vi "pupilometria_IR.vi"() -> ()   [LabVIEW 2024]
uses:
  <vilib>/vision/NI_Vision_Development_Module.lvlib
panel:
  out "Gray Image":T1(plugin-control)
  out "ROI manual":T1(plugin-control)
  out "error out":errorcluster
  in  "stop":bool
  out "Image Out":T1(plugin-control)
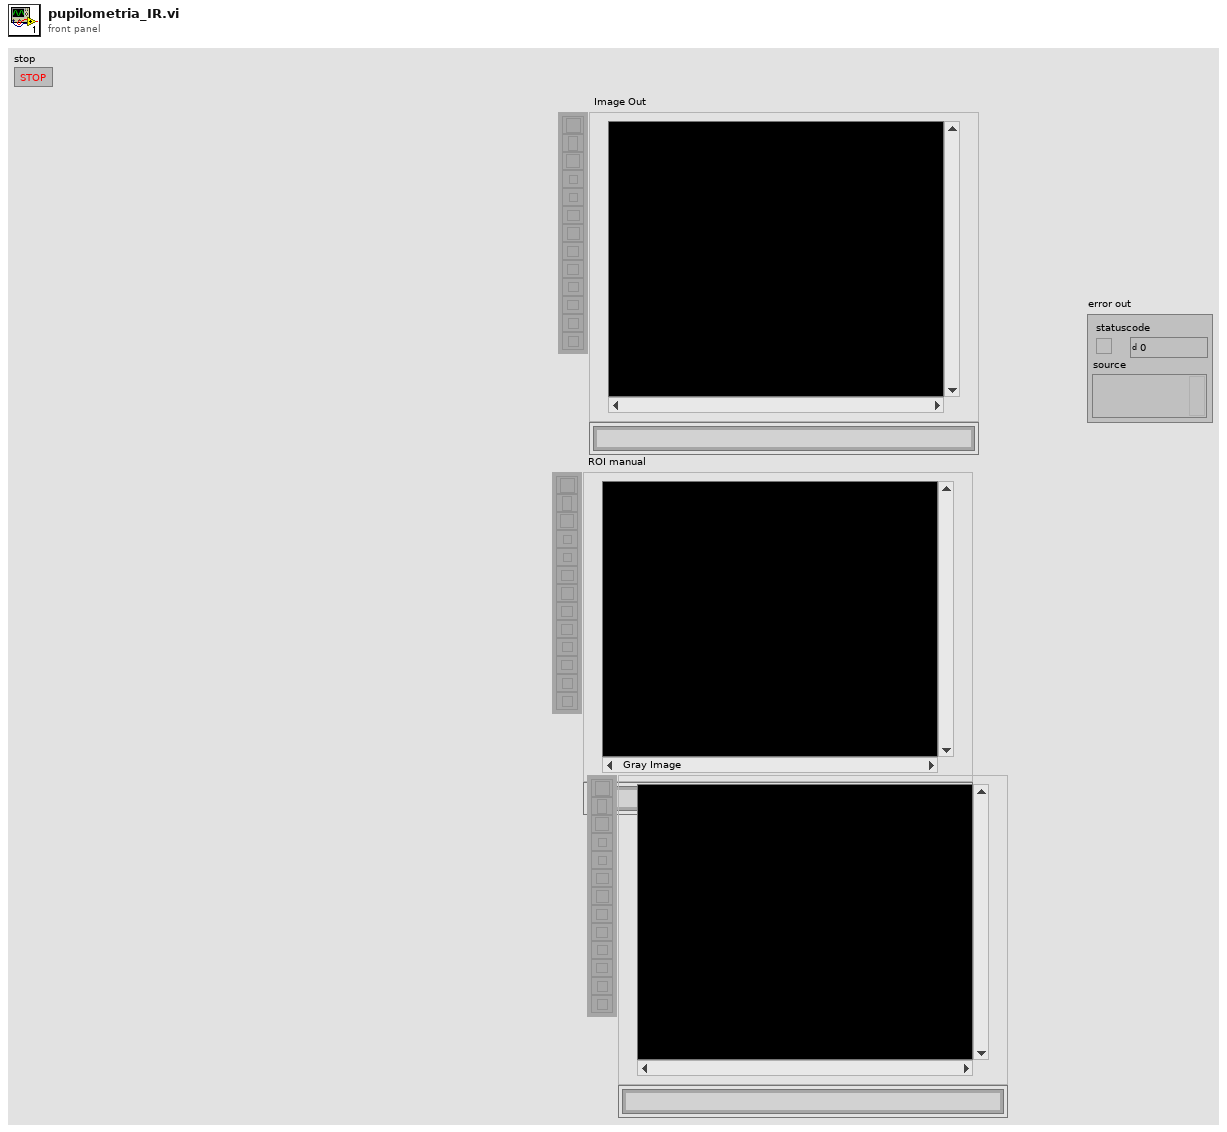
[diagram p1: front panel]
types:
  T1 = typedef "IMAQ Image.ctl" = refnum<image>
  T2 = typedef "Image Type" = u32
  T3 = cluster{"Global Rectangle":i32[], "Contours":cluster{"Contour Type":u32, "ROI Type":u32, "Points":i32[]}[]}
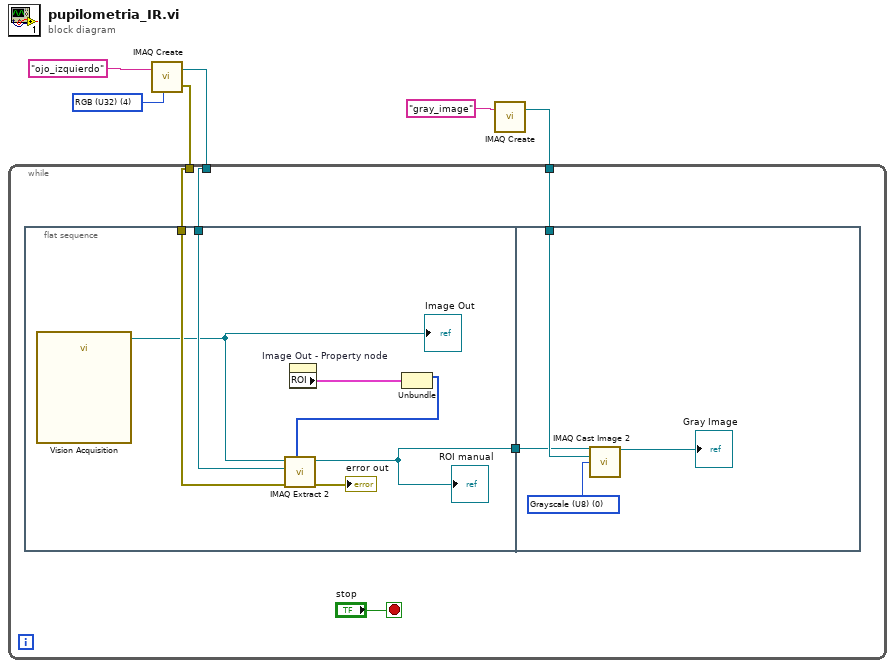
[diagram p0: block diagram]
diagram:
  w5 = T2 4 items=["Grayscale (U8)", "Grayscale (I16)", "Grayscale (SGL)", "Complex (CSG)", "RGB (U32)", "HSL (U32)", "RGB (U64)", "Grayscale (U16)"] ("Image Type")
  n1 = call "IMAQ Create"("Image Name"="ojo_izquierdo", "Image Type"=w5) -> ("New Image"=w3:T1, "error out"=w4:errorcluster)  [unwired: 3 in]
  n2 = call "IMAQ Create"("Image Name"="gray_image") -> ("New Image"=w1:T1)  [unwired: 4 in, 1 out]
  n3 = while {
    tunnel: w4 -> [w10]
    tunnel: w3 -> [w9]
    tunnel: w1 -> [w8]
    stop <- "stop" stop-if-true
    n4 = flat-sequence {
      tunnel: w10 -> [w15]
      tunnel: w9 -> [w14]
      tunnel: [w12] -> w7
      tunnel: w8 -> [w22]
      tunnel: w7 -> [w21]
      frame #0 {
        n5 = call "Vision Acquisition"() -> ("Image Out"=w13:T1)  [unwired: 25 in, 2 out]
        "Image Out" <- w13
        n6 = property on="Image Out - Property node" class="ImageControl"() -> ("ROI"=w18:T3)  [unwired: 2 in, 2 out]
        n7 = Unbundle "Unbundle"(w18) -> ("Global Rectangle"=w17:i32[])  [unwired: 1 out]
        n8 = call "IMAQ Extract 2"("Optional Rectangle"=w17, "error in (no error)"=w15, "Image Dst"=w14, "Image Src"=w13) -> ("error out"=→"error out":errorcluster, "Image Dst Out"=w12:T1)  [unwired: 6 in]
        "ROI manual" <- w12
      }
      frame #1 {
        w20 = T2 0 items=["Grayscale (U8)", "Grayscale (I16)", "Grayscale (SGL)", "Complex (CSG)", "RGB (U32)", "HSL (U32)", "RGB (U64)", "Grayscale (U16)"] ("Image Type")
        n9 = call "IMAQ Cast Image 2"("Image Src"=w21, "Image Dst"=w22, "Image Type"=w20) -> ("Image Dst Out"=→"Gray Image":T1)  [unwired: 11 in, 1 out]
      }
    }
  }
